vi "p35_1quaternion.vi"() -> ()   [LabVIEW 2013]
uses:
  <vilib>/Analysis/Matrix/Datatypes/RealMatrix.ctl
  <vilib>/robotics/Kinematics/Quaternion.ctl
  <vilib>/robotics/Kinematics/Divide Quaternion by Quaternion.vi
  <vilib>/Analysis/baseanly.llb/Outer Product.vi
  <vilib>/Analysis/baseanly.llb/Real Outer Product.vi
  <vilib>/robotics/Kinematics/Create Lie Group Matrix.vi
  <vilib>/robotics/Kinematics/Inverse Quaternion.vi
  <vilib>/Analysis/_algsub.llb/Vector Norm.vi
  <vilib>/Analysis/_algsub.llb/Real Vector Norm.vi
  <vilib>/Analysis/baseanly.llb/Dot Product.vi
  <vilib>/Analysis/baseanly.llb/Real Dot Product.vi
  <vilib>/robotics/Kinematics/Multiply Quaternion by Quaternion.vi
  <vilib>/robotics/Kinematics/Rotation Matrix to Angle Vector.vi
  <vilib>/Analysis/Matrix/Numeric/Multiply/Multiply.vi
  <vilib>/Analysis/Matrix/Numeric/Multiply/Multiply - RM,R.vi
  <vilib>/Analysis/Matrix/Numeric/Multiply/Multiply - R,RM.vi
  <vilib>/Analysis/Matrix/Numeric/Add/Add.vi
  <vilib>/Analysis/Matrix/Numeric/Add/Add - RM,RM.vi
  <vilib>/robotics/Kinematics/NI_Kinematics.lvlib
  <vilib>/Analysis/Matrix/NI_Matrix.lvlib
panel:
  out "rotation matrix":T1
  out "rotated vector":dbl[](array[numeric])
  out "transformation matrix":picture
  out "3D Picture":refnum<vi>(3d-picture)
  out "q * q~":dbl[](array[numeric])=[1.0, 1.0, 1.0] format="%#.3f"
  out "q / q":dbl[](array[numeric])=[1.0, 1.0, 1.0] format="%#.3f"
  out "Normalized quaternion":dbl
  out "3D Picture":refnum<vi>(3d-picture)
  out "Conjugate (q~)":dbl[](array[numeric])=[1.0, 1.0, 1.0]
  out "Quaternion":dbl[](array[numeric])=[1.0, 1.0, 1.0]
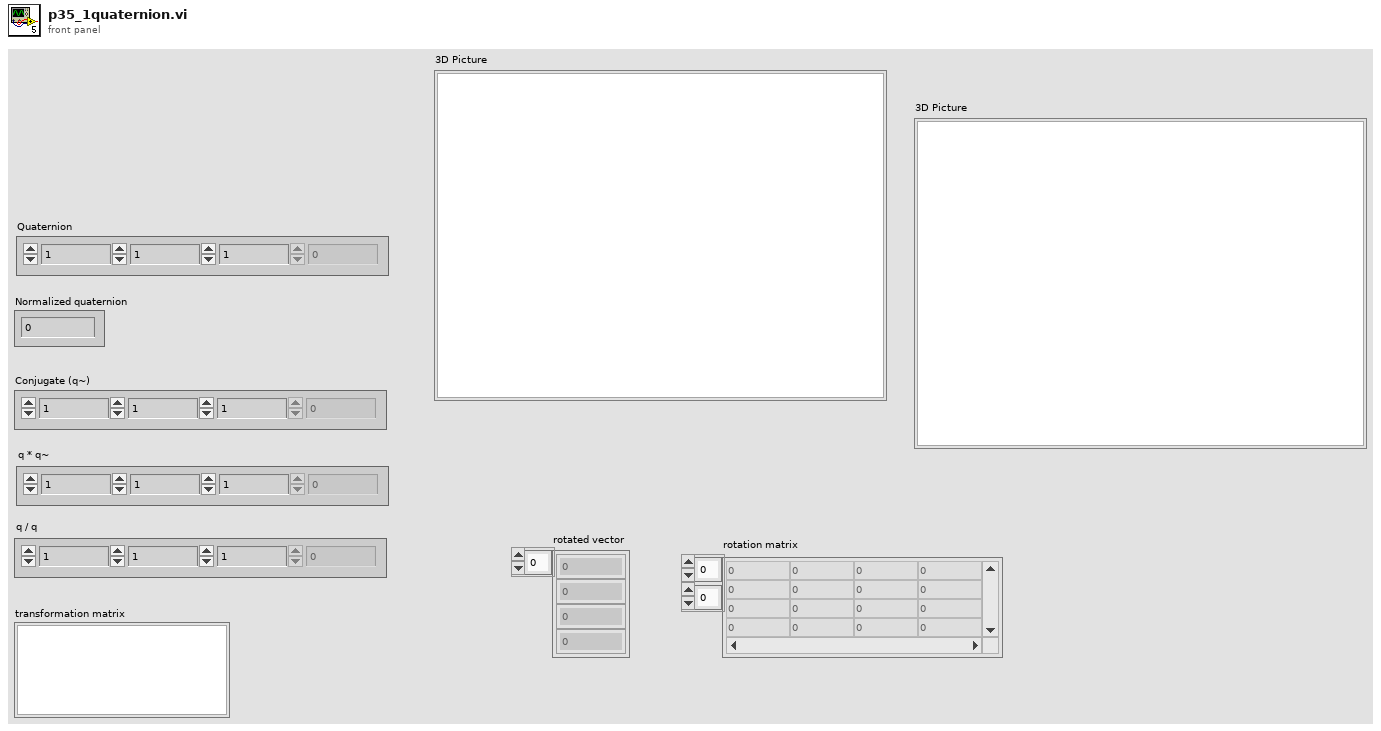
[diagram p1: front panel]
types:
  T1 = typedef "NI_Matrix.lvlib/RealMatrix.ctl" = dbl[][]
  T2 = typedef "NI_Kinematics.lvlib/Quaternion.ctl" = dbl[]
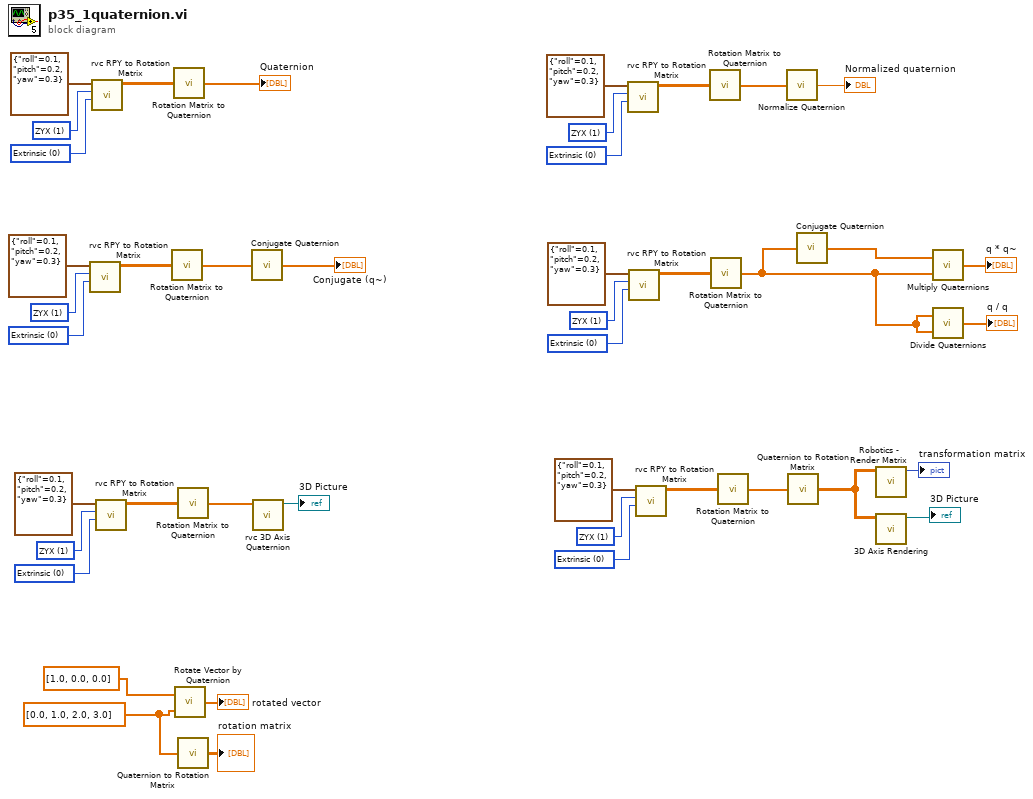
[diagram p0: block diagram]
diagram:
  w2 = T2 [0.0, 1.0, 2.0, 3.0] ("quaternion")
  w8 = u16 1 items=["XYZ", "ZYX"] ("Convension")
  w7 = u16 0 items=["Extrinsic", "Intrinsic"] ("type of rotations")
  w15 = u16 1 items=["XYZ", "ZYX"] ("Convension")
  w16 = u16 0 items=["Extrinsic", "Intrinsic"] ("type of rotations")
  w25 = u16 1 items=["XYZ", "ZYX"] ("Convension")
  w24 = u16 0 items=["Extrinsic", "Intrinsic"] ("type of rotations")
  w27 = u16 1 items=["XYZ", "ZYX"] ("Convension")
  w28 = u16 0 items=["Extrinsic", "Intrinsic"] ("type of rotations")
  w33 = u16 1 items=["XYZ", "ZYX"] ("Convension")
  w34 = u16 0 items=["Extrinsic", "Intrinsic"] ("type of rotations")
  w41 = u16 1 items=["XYZ", "ZYX"] ("Convension")
  w40 = u16 0 items=["Extrinsic", "Intrinsic"] ("type of rotations")
  n1 = call "rvc RPY to Rotation Matrix.vi"("type of rotations"=w28, "Convension"=w27, "angles"=cluster{"roll":dbl, "pitch":dbl, "yaw":dbl} {"roll"=0.1, "pitch"=0.2, "yaw"=0.3}) -> ("rotation matrix"=w30:T1)  [unwired: 8 in]
  n2 = call "rvc RPY to Rotation Matrix.vi"("type of rotations"=w40, "Convension"=w41, "angles"=cluster{"roll":dbl, "pitch":dbl, "yaw":dbl} {"roll"=0.1, "pitch"=0.2, "yaw"=0.3}) -> ("rotation matrix"=w38:T1)  [unwired: 8 in]
  n3 = call "rvc RPY to Rotation Matrix.vi"("type of rotations"=w16, "Convension"=w15, "angles"=cluster{"roll":dbl, "pitch":dbl, "yaw":dbl} {"roll"=0.1, "pitch"=0.2, "yaw"=0.3}) -> ("rotation matrix"=w14:T1)  [unwired: 8 in]
  n4 = call <vilib>:"Rotation Matrix to Quaternion.vi"("rotation matrix"=w30) -> ("quaternion"=w26:T2)
  n5 = call <vilib>:"Rotation Matrix to Quaternion.vi"("rotation matrix"=w38) -> ("quaternion"=→"Quaternion":T2)
  n6 = call <vilib>:"Rotate Vector by Quaternion.vi"("quaternion"=w2, "vector"=dbl[] [1.0, 0.0, 0.0]) -> ("rotated vector"=→"rotated vector":dbl[])  [unwired: 1 in]
  n7 = call <vilib>:"Rotation Matrix to Quaternion.vi"("rotation matrix"=w14) -> ("quaternion"=w13:T2)
  n8 = call <vilib>:"Quaternion to Rotation Matrix.vi"("quaternion"=w2) -> ("rotation matrix"=→"rotation matrix":T1)
  n9 = call <vilib>:"Conjugate Quaternion.vi"("quaternion"=w26) -> ("conjugate"=→"Conjugate (q~)":T2)
  n10 = call "rvc 3D Axis Quaternion.vi"("quaternion"=w13) -> ("SceneNode out"=→"3D Picture":refnum<vi>)  [unwired: 10 in]
  n11 = call "rvc RPY to Rotation Matrix.vi"("type of rotations"=w34, "Convension"=w33, "angles"=cluster{"roll":dbl, "pitch":dbl, "yaw":dbl} {"roll"=0.1, "pitch"=0.2, "yaw"=0.3}) -> ("rotation matrix"=w36:T1)  [unwired: 8 in]
  n12 = call "rvc RPY to Rotation Matrix.vi"("type of rotations"=w24, "Convension"=w25, "angles"=cluster{"roll":dbl, "pitch":dbl, "yaw":dbl} {"roll"=0.1, "pitch"=0.2, "yaw"=0.3}) -> ("rotation matrix"=w22:T1)  [unwired: 8 in]
  n13 = call "rvc RPY to Rotation Matrix.vi"("type of rotations"=w7, "Convension"=w8, "angles"=cluster{"roll":dbl, "pitch":dbl, "yaw":dbl} {"roll"=0.1, "pitch"=0.2, "yaw"=0.3}) -> ("rotation matrix"=w9:T1)  [unwired: 8 in]
  n14 = call <vilib>:"Rotation Matrix to Quaternion.vi"("rotation matrix"=w36) -> ("quaternion"=w31:T2)
  n15 = call <vilib>:"Rotation Matrix to Quaternion.vi"("rotation matrix"=w22) -> ("quaternion"=w18:T2)
  n16 = call <vilib>:"Rotation Matrix to Quaternion.vi"("rotation matrix"=w9) -> ("quaternion"=w11:T2)
  n17 = call <vilib>:"Normalize Quaternion.vi"("quaternion"=w31) -> ("normalized quaternion"=→"Normalized quaternion":dbl)
  n18 = call <vilib>:"Quaternion to Rotation Matrix.vi"("quaternion"=w11) -> ("rotation matrix"=w12:T1)
  n19 = call <vilib>:"Conjugate Quaternion.vi"("quaternion"=w18) -> ("conjugate"=w21:T2)
  n20 = call "Robotics - Render Matrix.vi"("A"=w12) -> ("picture out"=→"transformation matrix":picture)  [unwired: 10 in]
  n21 = call "3D Axis Rendering.vi"("rotation matrix"=w12) -> ("SceneNode out"=→"3D Picture":refnum<vi>)  [unwired: 9 in, 1 out]
  n22 = call-poly <vilib>:"Multiply Quaternions.vi"("y"=w18, "quaternion"=w21) -> ("product"=→"q * q~":T2)
  n23 = call-poly <vilib>:"Divide Quaternions.vi"("y"=w18, "quaternion"=w18) -> ("quotient"=→"q / q":T2)
